vi "4Pi Objective Image Alignment.vi"(7 "Calling VI Ref":refnum<vi>) -> ()   [LabVIEW 2016]
uses:
  4Pi OIA - Controls/4Pi OIA - ROI Selection.ctl
  4Pi OIA - Controls/4Pi OIA - Method.ctl
  <vilib>/vision/Image Controls.llb/IMAQ Image.ctl
  4Pi OIA - Controls/4Pi OIA - Notifier Type.ctl
  4Pi OIA - Controls/4Pi OIA - Actions.ctl
  <vilib>/Utility/miscctls.llb/LVPointTypeDef.ctl
  Hardware Configuration/Hardware Configuration Controls/Device Function.ctl
  Hardware Configuration/Hardware Configuration Controls/Device Type.ctl
  Device Library/Cameras/Hamamatsu/Orca Flash/Orca Flash Controls/Orca Flash Actions.ctl
  Device Library/Shutters/Shutter Controls/Shutter Actions.ctl
  Device Library/Stages/Stages Controls/Stage Actions.ctl
  <resource>/objmgr/IMAQImage.rc
panel:
  in  "Alignment Cycles":u16=1 min=1 step=1
  in  "Get Shift":bool
  in  "Camera Px. Size (µm)":dbl=0.1 min=0.0 max=10.0
  in  "Frame Accums.":u16=1 min=1 step=1
  in  "Align":bool
  in  "Method":T1
  in  "Image Selection":i32(ring) items=["Quad 01", "Quad 02", "Quad 03", "Quad 04"]
  in  "ROI Selection":T2
  in  "Quit":bool
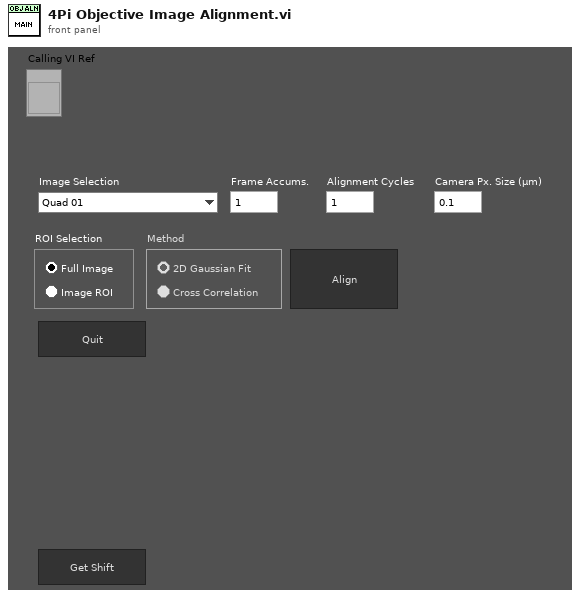
[diagram p1: front panel]
types:
  T1 = typedef "4Pi OIA - Method.ctl" = enum32{"2D Gaussian Fit", "Cross Correlation"}
  T2 = typedef "4Pi OIA - ROI Selection.ctl" = enum32{"Full Image", "ROI"}
  T3 = enum16{"Always On", "Always Off", "Off While Running"}
  T4 = typedef "LVPointTypeDef.ctl" = cluster{"Horizontal":i16, "Vertical":i16}
  T5 = typedef "4Pi OIA - Actions.ctl" = enum16{"Idle", "Start Alignment", "Get Upper Image", "Get Lower Image", "Get Shift", "Move OBJ", "Quit"}
  T6 = enum8{"Enabled", "Disabled", "Disabled and Grayed Out"}
  T7 = typedef "4Pi OIA - Notifier Type.ctl" = cluster{"Action":T5, "ROI Selection":T2, "Method":T1, "Frame Accums.":u16, "Camera Px. Size (µm)":dbl, "Image Ref":T8}
  T8 = typedef "IMAQ Image.ctl" = refnum<image>
  T9 = typedef "Device Function.ctl" = enum16{"Primary", "Secondary", "Overview", "Wide Field Drift Correction", "642 nm Excitation", "560 nm Excitation", "546 nm Excitation", "488 nm Excitation", "405 nm Excitation", "Objective Drift Correction", "Objective XY", "Objective Z", "Sample XY", "Sample Coarse Z", "Sample Z", "4Pi Lower", "4Pi Upper", "Adj Cavity"}
  T10 = typedef "Device Type.ctl" = enum16{"AOTF", "Camera", "Deformable Mirror", "Laser", "Shutter", "Stage"}
  T11 = typedef "Orca Flash Actions.ctl" = enum16{"IDLE", "PREVIEW", "RECORD", "Record Settings", "SETPARAM", "GETPARAM", "SETROI", "GETROI", "PROGRESSIVE MODE", "AREA MODE", "STATUS", "QUIT"}
  T12 = typedef "Shutter Actions.ctl" = enum16{"Open", "Close", "Toggle", "Status", "Quit"}
  T13 = typedef "Stage Actions.ctl" = enum16{"Get Position", "MVR", "MOVE", "HALT", "ONTARGET", "ERROR", "REFERENCE", "INIT", "VELOCITY", "STATUS", "EXIT", "HOME", "ZEROPOS", "NANOPOS", "ANALOG", "QUIT"}
  T14 = enum32{"Invalid", "Standard", "Closed", "Hidden", "Minimized", "Maximized"}
  T15 = typedef "2D Gaussian - Best Fit Parameters.ctl" = cluster{"Amplitude":dbl, "X Position":dbl, "Y Position":dbl, "X Width":dbl, "Y Width":dbl, "Offset":dbl}
  T16 = typedef "LVRectTypeDef.ctl" = cluster{"Left":i16, "Top":i16, "Right":i16, "Bottom":i16}
  T17 = typedef "LVBoundsTypeDef.ctl" = cluster{"Width":u32, "Height":u32}
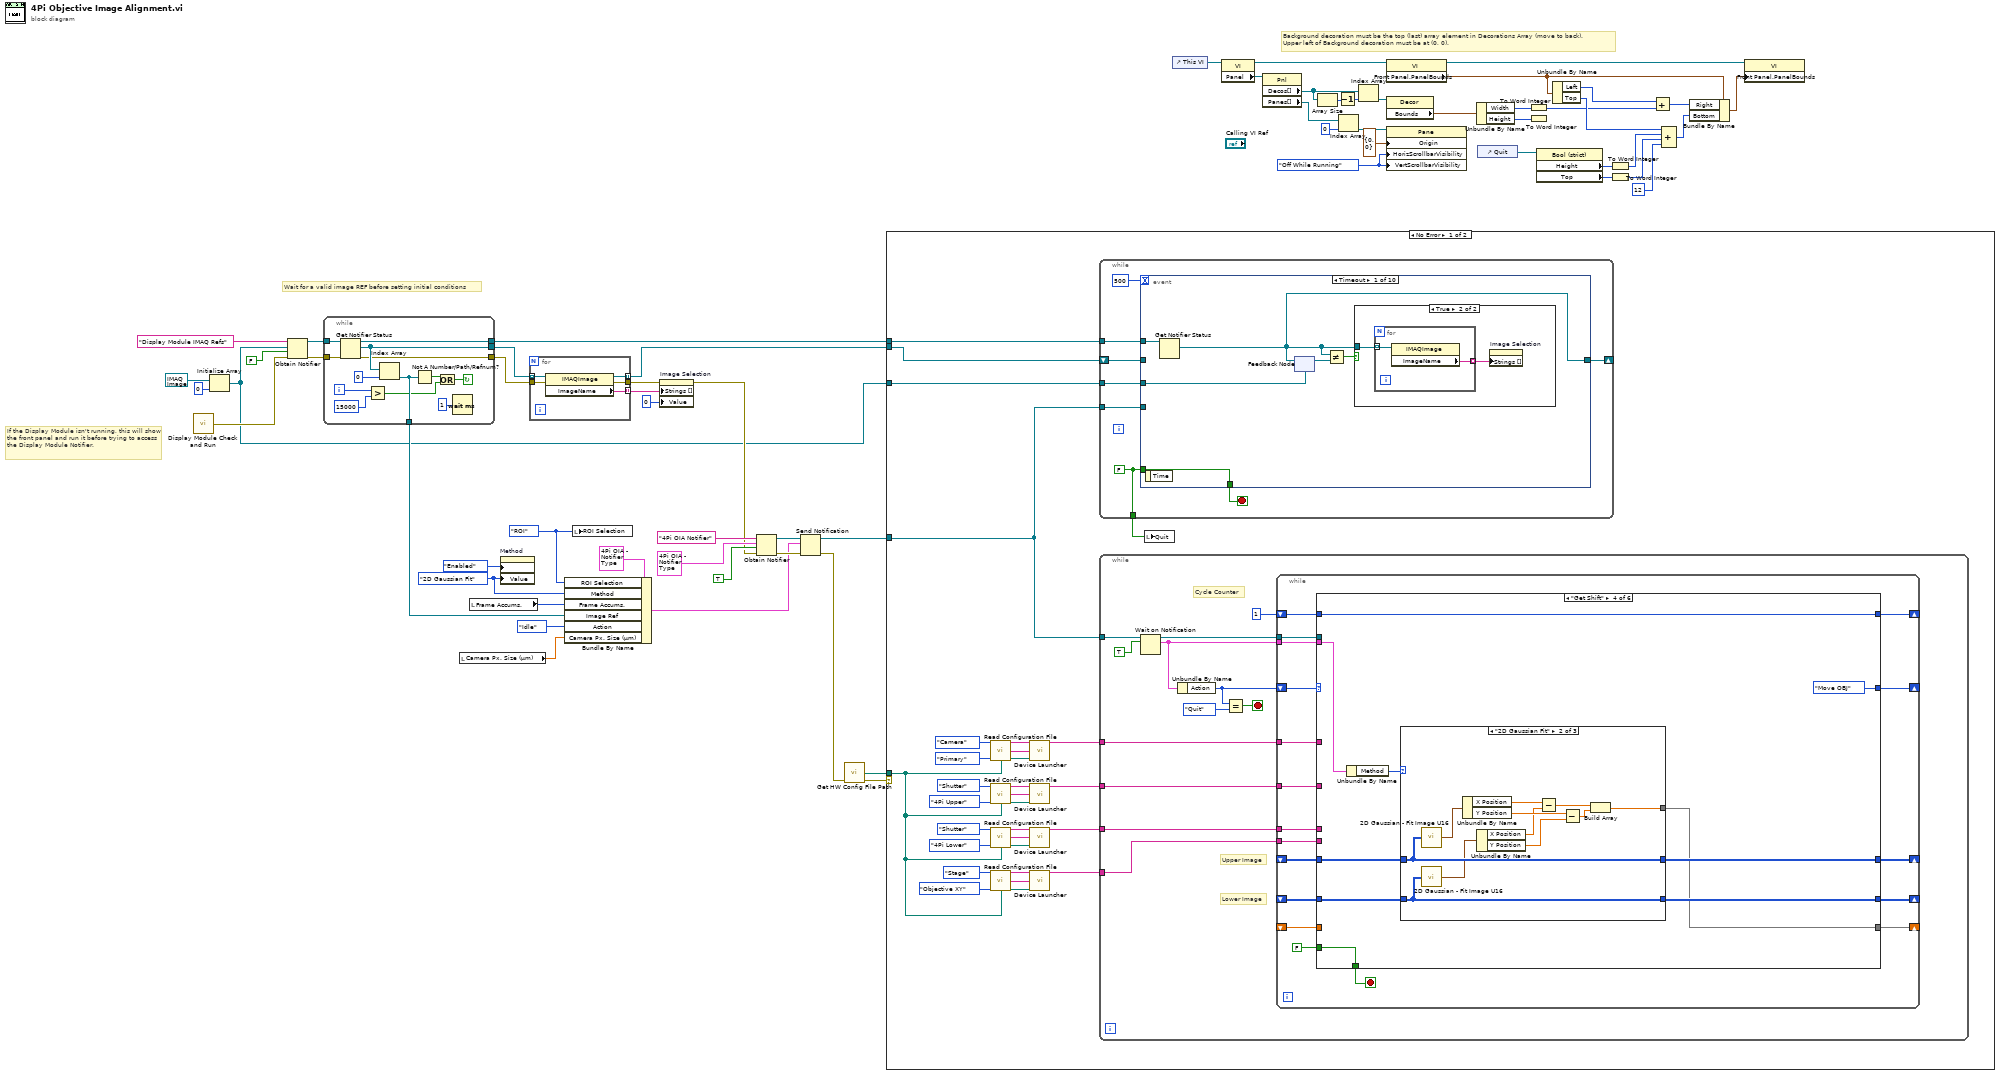
[diagram p0: block diagram]
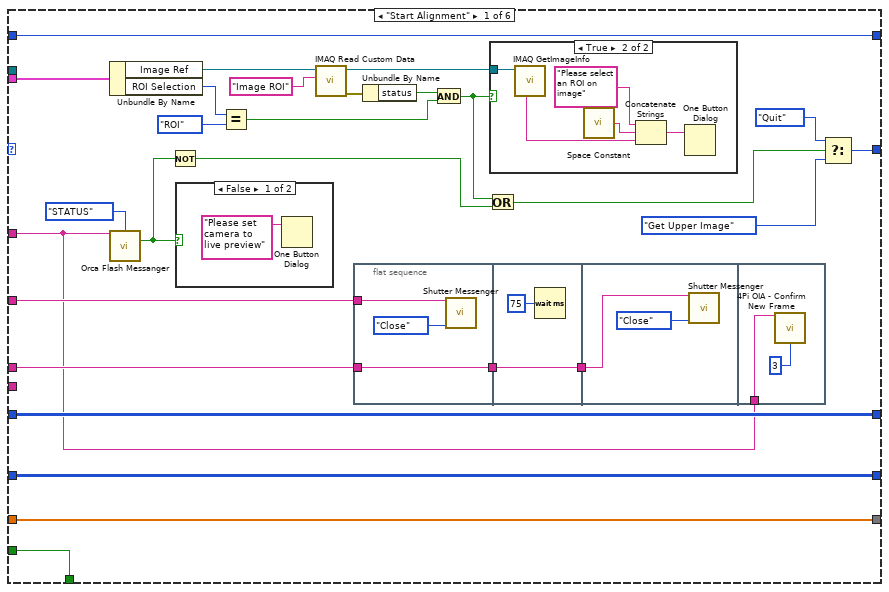
[diagram p2: hidden frame]
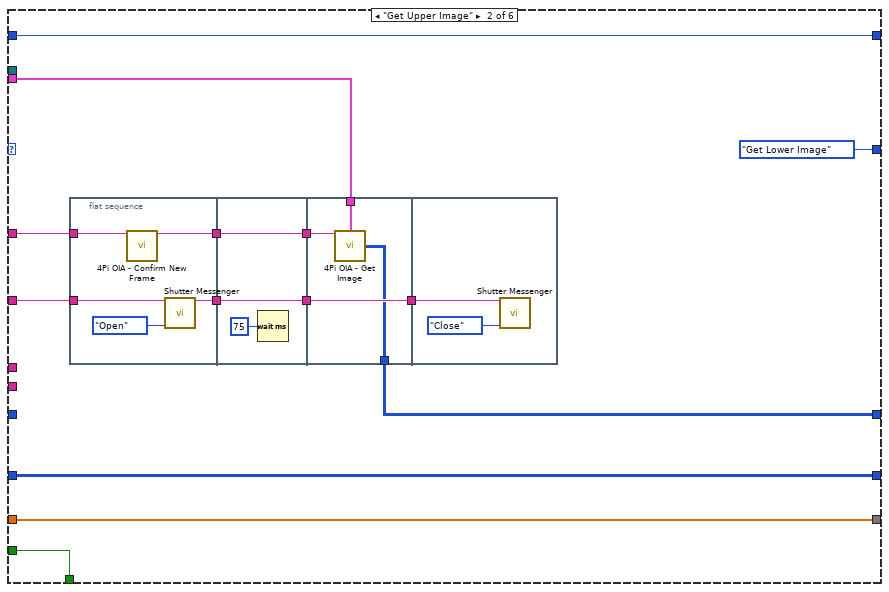
[diagram p5: hidden frame]
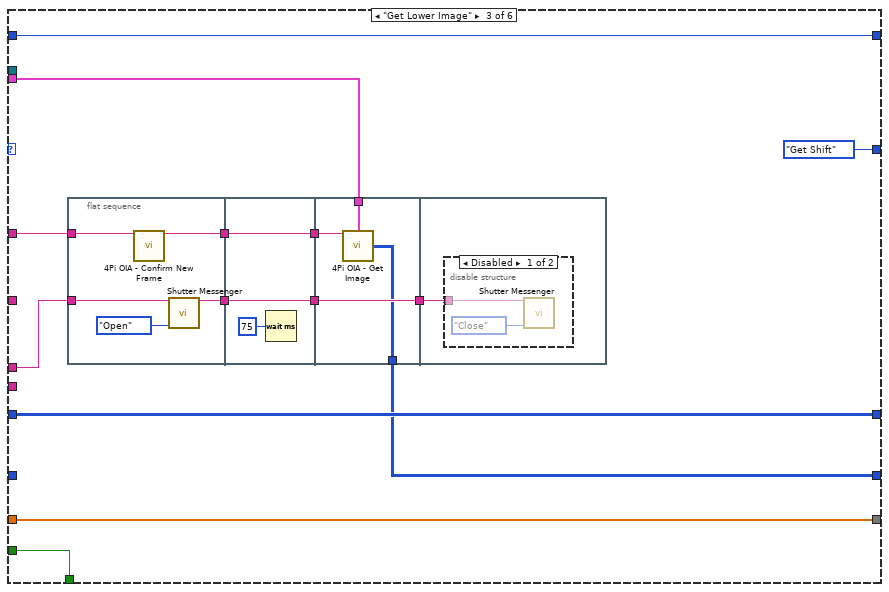
[diagram p6: hidden frame]
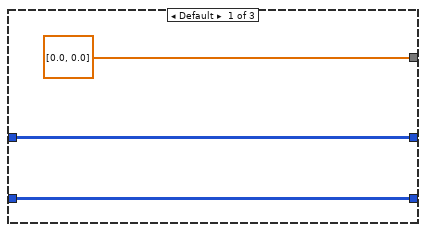
[diagram p8: hidden frame]
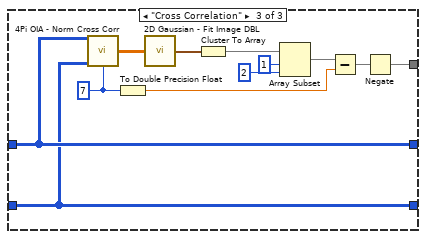
[diagram p9: hidden frame]
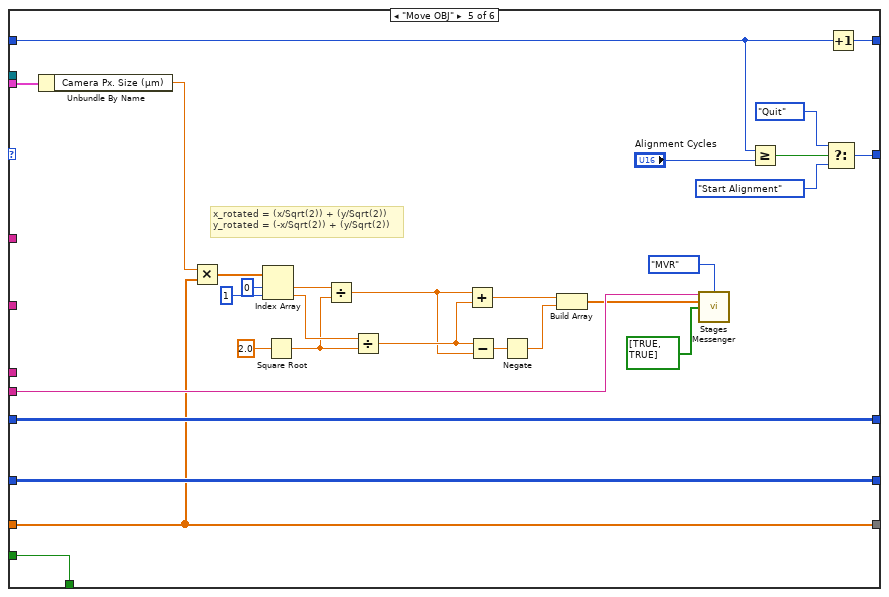
[diagram p10: hidden frame]
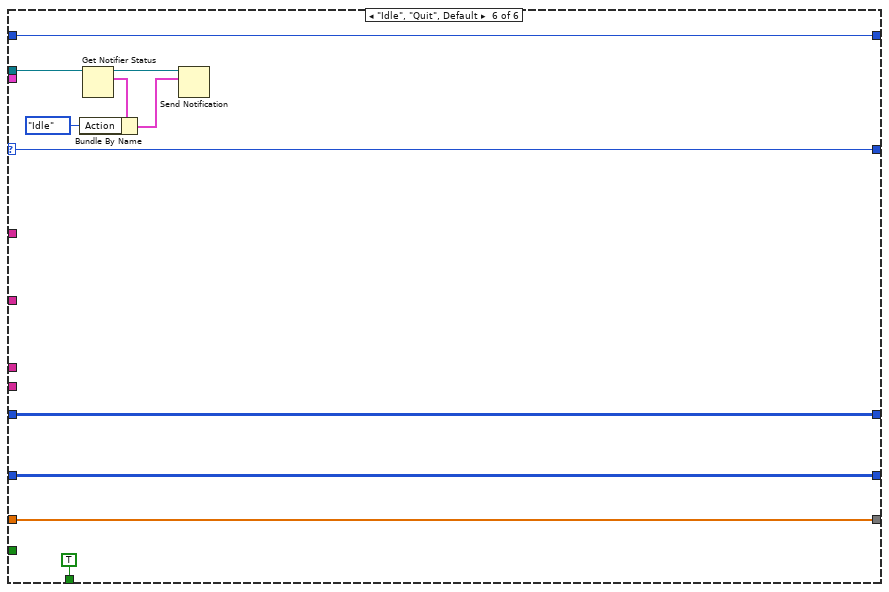
[diagram p11: hidden frame]
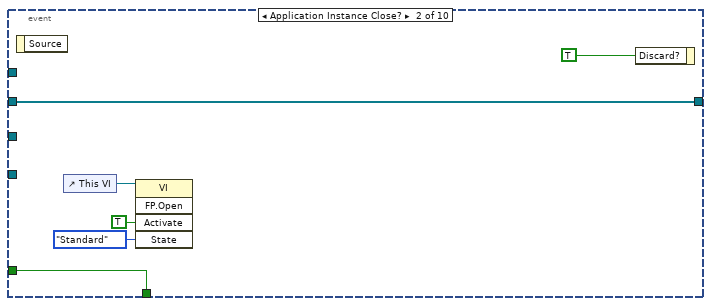
[diagram p13: hidden frame]
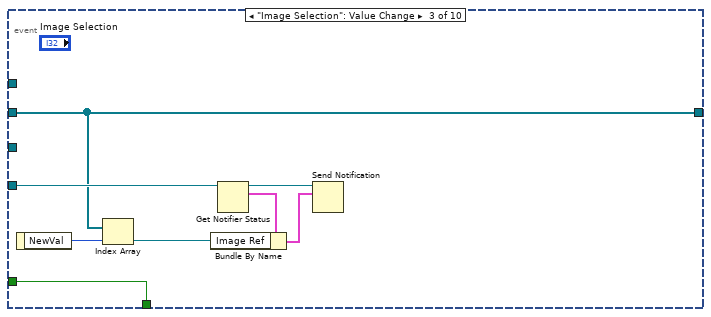
[diagram p14: hidden frame]
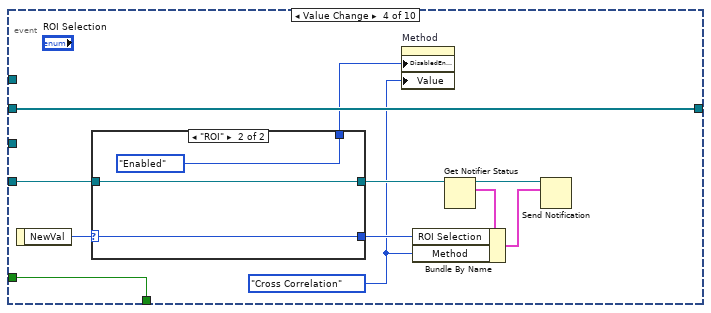
[diagram p15: hidden frame]
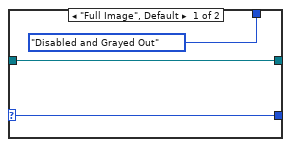
[diagram p16: hidden frame]
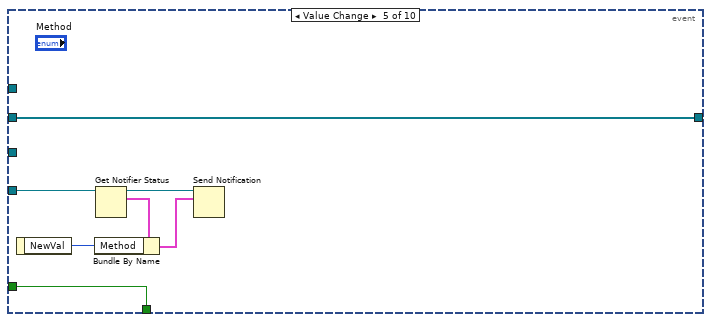
[diagram p17: hidden frame]
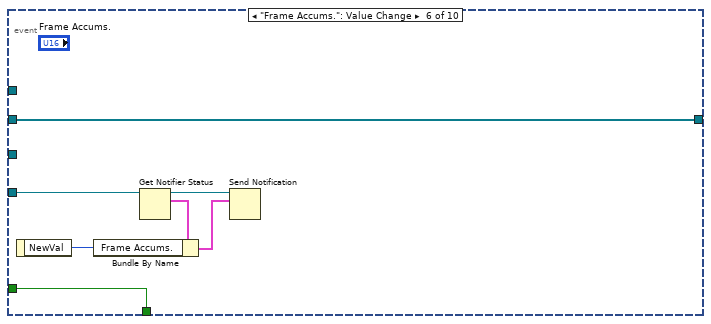
[diagram p18: hidden frame]
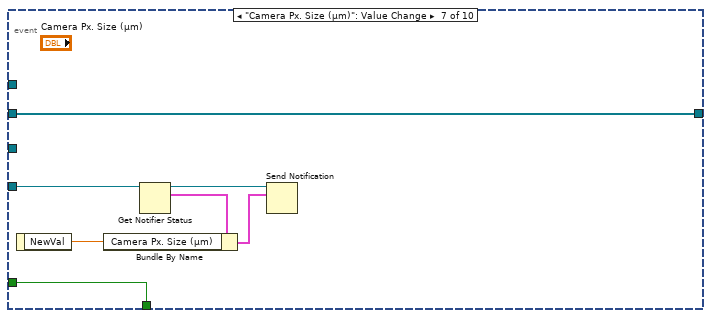
[diagram p19: hidden frame]
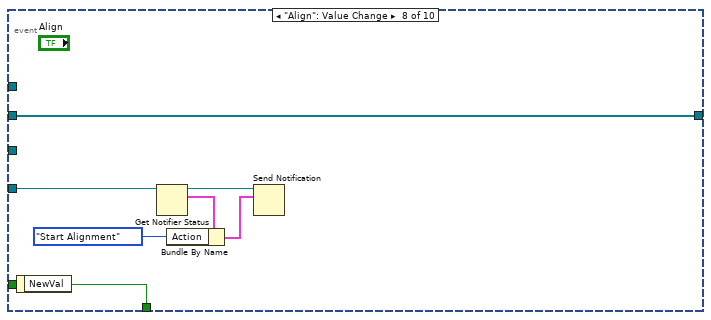
[diagram p20: hidden frame]
diagram:
  w25 = T3."Off While Running" ("Vertical Scrollbar Visibility")
  w51 = 4Pi_OIA_-_Method."2D Gaussian Fit" ("Method")
  w52 = 4Pi_OIA_-_ROI_Selection."ROI" ("ROI Selection")
  # "Wait for a valid image REF before setting initial conditions"
  # "If the Display Module isn't running, this will show the front panel and run it before trying to access the Display Module Notifier."
  # "Background decoration must be the top (last) array element in Decorations Array (move to back).\nUpper left of Background decoration must be at (0, 0)."
  n1 = call "Display Module Check and Run.vi"() -> ("Error"=w13:errorcluster)  [unwired: 15 in]
  n2 = Initialize Array(T8 refnum ("New Image"), 0 ("dimension size")) -> (w1:T8[])
  n3 = Obtain Notifier(name (unnamed)="Display Module IMAQ Refs", notification data type=w1, create if not found? (T)=FALSE, error in (no error)=w13) -> (notifier out=w12:refnum<notifier>, error out=w11:errorcluster)  [unwired: 1 out]
  n4 = while {
    tunnel: w12 -> [w76]
    tunnel: w11 -> [w75]
    tunnel: [w74] -> w10
    tunnel: [w73] -> w5
    tunnel: [w71] -> w9
    tunnel: [w69] -> w2
    i -> [w68]
    stop <- w65 continue-if-true
    n5 = Get Notifier Status(notifier=w76, error in (no error)=w75) -> (notifier out=w74:refnum<notifier>, current notification=w73:T8[], error out=w69:errorcluster)  [unwired: 2 out]
    n6 = Greater?(x=w68, y=15000) -> (0:w64:bool)
    n7 = Index Array(array=w73, index=0) -> (element=w71:T8)
    n8 = Not A Number/Path/Refnum?(number/path/refnum=w71) -> (NaN/Path/Refnum?=w66:bool)
    n9 = Or(x=w66, y=w64) -> (x .or. y?=w65:bool)
    n10 = Wait (ms)(milliseconds to wait=u32 1) -> ()  [unwired: 1 out]
  }
  n11 = local read "Camera Px. Size (µm)"() -> (w43:dbl)
  n12 = local read "Frame Accums."() -> (w45:u16)
  n13 = property on="Method" class="RadioBtnsControl (strict)"("DisabledEnum"=T6."Enabled" ("Disabled"), "Value"=w51) -> ()  [unwired: 2 in, 2 out]
  n14 = for {
    tunnel: w5 -> [w81] mode=indexing
    tunnel: [w80] -> w8 mode=indexing
    tunnel: [w79] -> w6
    tunnel: [w78] -> w4 mode=indexing
    tunnel: w2 -> [w77]
    n15 = property class="IMAQImage"(reference=w81, error in=w77) -> (reference out=w78:T8, error out=w79:errorcluster, "ImageName"=w80:string)
  }
  n16 = Bundle By Name(cluster=T7 {"Action"=enum."Start Alignment", "ROI Selection"=enum."Full Image", "Method"=enum."2D Gaussian Fit", "Frame Accums."=0, "Camera Px. Size (µm)"=0.0, "Image Ref"=refnum} ("4Pi OIA Notifier Type"), "ROI Selection"=w52, "Method"=w51, "Frame Accums."=w45, "Image Ref"=w9, "Action"=4Pi_OIA_-_Actions."Idle", "Camera Px. Size (µm)"=w43) -> (w47:T7)
  n17 = local write "ROI Selection"(w52) -> ()
  n18 = property on="Image Selection" class="Ring (strict)"(error in=w6, "Strings []"=w8, "Value"=0) -> (error out=w3:errorcluster)  [unwired: 1 in, 1 out]
  n19 = Obtain Notifier(name (unnamed)="4Pi OIA Notifier", notification data type=T7 {"Action"=enum."Start Alignment", "ROI Selection"=enum."Full Image", "Method"=enum."2D Gaussian Fit", "Frame Accums."=0, "Camera Px. Size (µm)"=0.0, "Image Ref"=refnum} ("4Pi OIA Notifier Type"), create if not found? (T)=TRUE, error in (no error)=w3) -> (notifier out=w50:refnum<notifier>, error out=w48:errorcluster)  [unwired: 1 out]
  n20 = Send Notification(notification=w47, notifier=w50, error in (no error)=w48) -> (notifier out=w49:refnum<notifier>, error out=w46:errorcluster)
  n21 = call "Get HW Config File Path.vi"("Error"=w46) -> ("File Path"=w62:path, "Error"=w63:errorcluster)  [unwired: 13 in]
  n22 = case shown="No Error" w63 {
    tunnel: w62 -> [w110 _]
    tunnel: w10 -> [w109 _]
    tunnel: w1 -> [w108 _]
    tunnel: w49 -> [w106 _]
    tunnel: w4 -> [w107 _]
    frame No Error {
      n23 = call "Read Configuration File.vi"("Device Type"=Device_Type."Camera", "Device Function"=Device_Function."Primary", "Config File Path"=w110) -> ("Unique Notifier Name"=w100:string, "Device Ports/IDs/Channels"=w102:string[], "Device Engine Path"=w101:path)  [unwired: 9 in, 1 out]
      n24 = call "Read Configuration File.vi"("Device Type"=Device_Type."Shutter", "Device Function"=Device_Function."4Pi Upper", "Config File Path"=w110) -> ("Unique Notifier Name"=w85:string, "Device Ports/IDs/Channels"=w87:string[], "Device Engine Path"=w86:path)  [unwired: 9 in, 1 out]
      n25 = call "Read Configuration File.vi"("Device Type"=Device_Type."Shutter", "Device Function"=Device_Function."4Pi Lower", "Config File Path"=w110) -> ("Unique Notifier Name"=w90:string, "Device Ports/IDs/Channels"=w88:string[], "Device Engine Path"=w89:path)  [unwired: 9 in, 1 out]
      n26 = call "Read Configuration File.vi"("Device Type"=Device_Type."Stage", "Device Function"=Device_Function."Objective XY", "Config File Path"=w110) -> ("Unique Notifier Name"=w95:string, "Device Ports/IDs/Channels"=w97:string[], "Device Engine Path"=w96:path)  [unwired: 9 in, 1 out]
      n27 = call "Device Launcher.vi"("Notifier Name"=w100, "Device Ports/IDs/Channels"=w102, "Device Engine Path"=w101) -> ("Notifier Name"=w105:string)  [unwired: 11 in, 1 out]
      n28 = call "Device Launcher.vi"("Notifier Name"=w85, "Device Ports/IDs/Channels"=w87, "Device Engine Path"=w86) -> ("Notifier Name"=w104:string)  [unwired: 11 in, 1 out]
      n29 = call "Device Launcher.vi"("Notifier Name"=w90, "Device Ports/IDs/Channels"=w88, "Device Engine Path"=w89) -> ("Notifier Name"=w103:string)  [unwired: 11 in, 1 out]
      n30 = call "Device Launcher.vi"("Notifier Name"=w95, "Device Ports/IDs/Channels"=w97, "Device Engine Path"=w96) -> ("Notifier Name"=w82:string)  [unwired: 11 in, 1 out]
      n31 = while {
        tunnel: [w322] -> w111
        tunnel: w109 -> [w321]
        tunnel: w108 -> [w320]
        tunnel: w106 -> [w319]
        shift-right: [w318] -> _
        shift-left: w107 -> [w317]
        stop <- w323 stop-if-true
        w322 = FALSE
        n32 = event shown="[0] Timeout" {
          selector: _ -> [_ _ _ _ _ _ _ _ _ _]
          dyn-events: _ -> [_ _ _ _ _ _ _ _ _ _]
          timeout: 500 -> [_ _ _ _ _ _ _ _ _ _]
          tunnel: w322 -> [w330 w339 w348 w358 w372 w379 w386 w393 w400 _]
          tunnel: [w330 w339 w348 w358 w372 w379 w386 w393 w400 w407] -> w323
          tunnel: w321 -> [w329 _ _ _ _ _ _ _ _ _]
          tunnel: w320 -> [w328 _ _ _ _ _ _ _ _ _]
          tunnel: w319 -> [_ _ w347 w353 w367 w374 w381 w392 w399 w401]
          tunnel: [w327 w335 w341 w359 w371 w378 w385 w387 w394 w406] -> w318
          tunnel: w317 -> [_ w335 w341 w359 w371 w378 w385 w387 w394 w406]
          event Timeout {
            n33 = event-data() -> ()  [unwired: 1 in, 1 out]
            n34 = Get Notifier Status(notifier=w329) -> (current notification=w327:T8[])  [unwired: 1 in, 4 out]
            n35 = feedback #1(w328) -> (w326:T8[])
            n36 = feedback-in #1(w327) -> ()
            n37 = Not Equal?(x=w327, y=w326) -> (x != y?=w325:bool)
            n38 = case shown="True" w325 {
              tunnel: w327 -> [_ w332]
              frame False {
              }
              frame True {
                n39 = for {
                  tunnel: w332 -> [w334] mode=indexing
                  tunnel: [w333] -> w331 mode=indexing
                  n40 = property class="IMAQImage"(reference=w334) -> ("ImageName"=w333:string)  [unwired: 1 in, 2 out]
                }
                n41 = property on="Image Selection" class="Ring (strict)"("Strings []"=w331) -> ()  [unwired: 2 in, 2 out]
              }
            }
          }
          event Application Instance Close? {
            n42 = event-data() -> ()  [unwired: 1 in, 1 out]
            n43 = control-ref of="This VI"() -> (w336:refnum<vi>)
            n44 = invoke class="VI" method="FP.Open"(reference=w336, "Activate"=TRUE ("Activate?"), "State"=T14."Standard") -> ()  [unwired: 2 in, 5 out]
            n45 = event-data("Discard?"=TRUE) -> ()  [unwired: 1 in, 1 out]
          }
          event "Image Selection": Value Change {
            n46 = event-data() -> ("NewVal"=w343:i32)  [unwired: 1 in]
            n47 = Index Array(array=w341, index=w343) -> (element=w342:T8)
            n48 = Get Notifier Status(notifier=w347) -> (notifier out=w346:refnum<notifier>, current notification=w345:T7)  [unwired: 1 in, 3 out]
            n49 = Bundle By Name(cluster=w345, "Image Ref"=w342) -> (w344:T7)
            n50 = Send Notification(notification=w344, notifier=w346) -> ()  [unwired: 1 in, 2 out]
          }
          event Value Change {
            w349 = 4Pi_OIA_-_Method."Cross Correlation" ("Method")
            n51 = event-data() -> ("NewVal"=w354:T2)  [unwired: 1 in]
            n52 = case shown="\"ROI\"" w354 {
              selector: w354 -> [w362 w364]
              tunnel: w353 -> [w361 w365]
              tunnel: [w362 w364] -> w351
              tunnel: [w361 w365] -> w352
              tunnel: [T6."Disabled and Grayed Out" ("Disabled") T6."Enabled" ("Disabled")] -> w350
              frame "Full Image", Default {
              }
              frame "ROI" {
              }
            }
            n53 = property on="Method" class="RadioBtnsControl (strict)"("DisabledEnum"=w350, "Value"=w349) -> ()  [unwired: 2 in, 2 out]
            n54 = Get Notifier Status(notifier=w352) -> (notifier out=w357:refnum<notifier>, current notification=w356:T7)  [unwired: 1 in, 3 out]
            n55 = Bundle By Name(cluster=w356, "ROI Selection"=w351, "Method"=w349) -> (w355:T7)
            n56 = Send Notification(notification=w355, notifier=w357) -> ()  [unwired: 1 in, 2 out]
          }
          event Value Change {
            n57 = event-data() -> ("NewVal"=w366:T1)  [unwired: 1 in]
            n58 = Get Notifier Status(notifier=w367) -> (notifier out=w370:refnum<notifier>, current notification=w369:T7)  [unwired: 1 in, 3 out]
            n59 = Bundle By Name(cluster=w369, "Method"=w366) -> (w368:T7)
            n60 = Send Notification(notification=w368, notifier=w370) -> ()  [unwired: 1 in, 2 out]
          }
          event "Frame Accums.": Value Change {
            n61 = event-data() -> ("NewVal"=w373:u16)  [unwired: 1 in]
            n62 = Get Notifier Status(notifier=w374) -> (notifier out=w377:refnum<notifier>, current notification=w376:T7)  [unwired: 1 in, 3 out]
            n63 = Bundle By Name(cluster=w376, "Frame Accums."=w373) -> (w375:T7)
            n64 = Send Notification(notification=w375, notifier=w377) -> ()  [unwired: 1 in, 2 out]
          }
          event "Camera Px. Size (µm)": Value Change {
            n65 = event-data() -> ("NewVal"=w380:dbl)  [unwired: 1 in]
            n66 = Get Notifier Status(notifier=w381) -> (notifier out=w384:refnum<notifier>, current notification=w383:T7)  [unwired: 1 in, 3 out]
            n67 = Bundle By Name(cluster=w383, "Camera Px. Size (µm)"=w380) -> (w382:T7)
            n68 = Send Notification(notification=w382, notifier=w384) -> ()  [unwired: 1 in, 2 out]
          }
          event "Align": Value Change {
            n69 = event-data() -> ()  [unwired: 1 in, 1 out]
            n70 = Get Notifier Status(notifier=w392) -> (notifier out=w391:refnum<notifier>, current notification=w390:T7)  [unwired: 1 in, 3 out]
            n71 = Bundle By Name(cluster=w390, "Action"=4Pi_OIA_-_Actions."Start Alignment") -> (w389:T7)
            n72 = Send Notification(notification=w389, notifier=w391) -> ()  [unwired: 1 in, 2 out]
          }
          event "Get Shift": Value Change {
            # "For debugging only"
            n73 = event-data() -> ()  [unwired: 1 in, 1 out]
            n74 = Get Notifier Status(notifier=w399) -> (notifier out=w398:refnum<notifier>, current notification=w397:T7)  [unwired: 1 in, 3 out]
            n75 = Bundle By Name(cluster=w397, "Action"=4Pi_OIA_-_Actions."Get Shift") -> (w396:T7)
            n76 = Send Notification(notification=w396, notifier=w398) -> ()  [unwired: 1 in, 2 out]
          }
          event "Quit": Value Change {
            n77 = event-data() -> ("NewVal"=w407:bool)  [unwired: 1 in]
            n78 = Get Notifier Status(notifier=w401) -> (notifier out=w402:refnum<notifier>, current notification=w403:T7)  [unwired: 1 in, 3 out]
            n79 = Bundle By Name(cluster=w403, "Action"=4Pi_OIA_-_Actions."Quit") -> (w404:T7)
            n80 = Send Notification(notification=w404, notifier=w402) -> ()  [unwired: 1 in, 2 out]
          }
        }
      }
      n81 = while {
        tunnel: w106 -> [w123]
        tunnel: w105 -> [w118]
        tunnel: w104 -> [w117]
        tunnel: w103 -> [w116]
        tunnel: w82 -> [w113]
        stop <- w120 stop-if-true
        # "Cycle Counter"
        # "Lower Image"
        # "Upper Image"
        n82 = Wait on Notification(notifier=w123, ignore previous (F)=TRUE) -> (notifier out=w114:refnum<notifier>, notification=w115:T7)  [unwired: 2 in, 2 out]
        n83 = Unbundle By Name(w115) -> ("Action"=w119:T5)
        n84 = Equal?(x=w119, y=4Pi_OIA_-_Actions."Quit") -> (x = y?=w120:bool)
        n85 = while {
          shift-right: [w138] -> _
          shift-left: w119 -> [w141]
          tunnel: w118 -> [w137]
          tunnel: w117 -> [w136]
          tunnel: w116 -> [w135]
          shift-right: [w132] -> _
          shift-left: _ -> [w131]
          shift-right: [w134] -> _
          shift-left: _ -> [w133]
          tunnel: w115 -> [w130]
          tunnel: w114 -> [w129]
          tunnel: w113 -> [w128]
          shift-right: [w127] -> _
          shift-left: _ -> [w126]
          shift-right: [w124] -> _
          shift-left: u16 1 -> [w125]
          stop <- w139 stop-if-true
          n86 = case shown="\"Get Shift\"" w141 {
            selector: w141 -> [_ _ _ _ _ w315]
            tunnel: FALSE -> [w168 w196 w224 w249 w305 _]
            tunnel: [w168 w196 w224 w249 w305 TRUE] -> w139
            tunnel: [w153 4Pi_OIA_-_Actions."Get Lower Image" ("Action") 4Pi_OIA_-_Actions."Get Shift" ("Action") 4Pi_OIA_-_Actions."Move OBJ" ("Action") w279 w315] -> w138
            tunnel: w137 -> [w145 w187 w218 _ _ _]
            tunnel: w136 -> [w151 w195 _ _ _ _]
            tunnel: w135 -> [w150 _ w215 _ _ _]
            tunnel: [w147 w189 w216 w243 w303 w313] -> w134
            tunnel: w133 -> [w147 w189 _ w245 w303 w313]
            tunnel: [w146 w188 w217 w244 w304 w314] -> w132
            tunnel: w131 -> [w146 _ w217 w246 w304 w314]
            tunnel: w130 -> [w144 w186 w214 w247 w299 _]
            tunnel: w129 -> [_ _ _ _ _ w308]
            tunnel: w128 -> [_ _ _ _ w302 _]
            tunnel: [w143 w185 w213 w242 w287 w307] -> w127
            tunnel: w126 -> [w143 w185 w213 _ w287 w307]
            tunnel: w125 -> [w142 w184 w212 w241 w278 w306]
            tunnel: [w142 w184 w212 w241 w277 w306] -> w124
            frame "Start Alignment" {
              n87 = Unbundle By Name(w144) -> ("Image Ref"=w165:T8, "ROI Selection"=w167:T2)
              n88 = call "Orca Flash Messanger.vi"("Notifier Name"=w145, "Camera Actions"=Orca_Flash_Actions."STATUS") -> ("Running?"=w157:bool)  [unwired: 9 in, 4 out]
              n89 = Not(x=w157) -> (.not. x?=w156:bool)
              n90 = case shown="False" w157 {
                frame False {
                  n91 = One Button Dialog(message="Please set camera to live preview") -> ()  [unwired: 1 in, 1 out]
                }
                frame True {
                }
              }
              n92 = Equal?(x=w167, y=4Pi_OIA_-_ROI_Selection."ROI") -> (x = y?=w161:bool)
              n93 = call "IMAQ Read Custom Data"("Key"="Image ROI", "Image"=w165) -> ("error out"=w163:errorcluster, "Image (duplicate)"=w160:T8)  [unwired: 7 in, 1 out]
              n94 = flat-sequence {
                tunnel: w151 -> [w170]
                tunnel: w150 -> [w169]
                tunnel: [w169] -> w149
                tunnel: w149 -> [w173]
                tunnel: [w173] -> w148
                tunnel: w148 -> [w174]
                tunnel: w145 -> [w177]
                frame #0 {
                  n95 = call "Shutter Messenger.vi"("Notifier Name"=w170, "Action"=Shutter_Actions."Close") -> ()  [unwired: 12 in, 2 out]
                }
                frame #1 {
                  n96 = Wait (ms)(milliseconds to wait=u32 75) -> ()  [unwired: 1 out]
                }
                frame #2 {
                  n97 = call "Shutter Messenger.vi"("Notifier Name"=w174, "Action"=Shutter_Actions."Close") -> ()  [unwired: 12 in, 2 out]
                }
                frame #3 {
                  n98 = call "4Pi OIA - Confirm New Frame.vi"("Camera Notifier Name"=w177, "Wait No. (1)"=u32 3 ("Wait No.")) -> ()  [unwired: 13 in, 1 out]
                }
              }
              n99 = Unbundle By Name(w163) -> ("status"=w162:bool)
              n100 = And(x=w162, y=w161) -> (x .and. y?=w158:bool)
              n101 = Or(x=w158, y=w156) -> (x .or. y?=w155:bool)
              n102 = case shown="True" w158 {
                tunnel: w160 -> [_ w183]
                frame False {
                }
                frame True {
                  n103 = call "IMAQ GetImageInfo"("Image"=w183) -> ("Image Name"=w182:string)  [unwired: 3 in, 7 out]
                  n104 = call <vilib>:"Space Constant.vi"() -> ("String"=w181:string)
                  n105 = Concatenate Strings("Please select an ROI on image", w181, w182) -> (w179:string)
                  n106 = One Button Dialog(message=w179) -> ()  [unwired: 1 in, 1 out]
                }
              }
              n107 = Select(t=4Pi_OIA_-_Actions."Quit" ("Action"), s=w155, f=4Pi_OIA_-_Actions."Get Upper Image") -> (s? t:f=w153:T5)
            }
            frame "Get Upper Image" {
              n108 = flat-sequence {
                tunnel: [w200] -> w192
                tunnel: [w198] -> w190
                tunnel: w195 -> [w201]
                tunnel: w187 -> [w199]
                tunnel: [w205] -> w193
                tunnel: w192 -> [w205]
                tunnel: [w203] -> w191
                tunnel: w190 -> [w203]
                tunnel: [w209] -> w194
                tunnel: w193 -> [w209]
                tunnel: w191 -> [w208]
                tunnel: w186 -> [w207]
                tunnel: [w206] -> w188
                tunnel: w194 -> [w210]
                frame #0 {
                  n109 = call "4Pi OIA - Confirm New Frame.vi"("Camera Notifier Name"=w199) -> ("Camera Notifier Name (Dup)"=w198:string)  [unwired: 14 in]
                  n110 = call "Shutter Messenger.vi"("Notifier Name"=w201, "Action"=Shutter_Actions."Open") -> ("Notifier Name Dup"=w200:string)  [unwired: 12 in, 1 out]
                }
                frame #1 {
                  n111 = Wait (ms)(milliseconds to wait=u32 75) -> ()  [unwired: 1 out]
                }
                frame #2 {
                  n112 = call "4Pi OIA - Get Image.vi"("Camera Notifier Name"=w208, "Alignment Data"=w207) -> ("Image Out"=w206:u16[][])  [unwired: 13 in]
                }
                frame #3 {
                  n113 = call "Shutter Messenger.vi"("Notifier Name"=w210, "Action"=Shutter_Actions."Close") -> ()  [unwired: 12 in, 2 out]
                }
              }
            }
            frame "Get Lower Image" {
              n114 = flat-sequence {
                tunnel: [w229] -> w221
                tunnel: [w226] -> w219
                tunnel: w218 -> [w227]
                tunnel: w215 -> [w228]
                tunnel: [w233] -> w222
                tunnel: w221 -> [w233]
                tunnel: [w231] -> w220
                tunnel: w219 -> [w231]
                tunnel: [w237] -> w223
                tunnel: w222 -> [w237]
                tunnel: w220 -> [w236]
                tunnel: w214 -> [w235]
                tunnel: [w234] -> w216
                tunnel: w223 -> [w238]
                frame #0 {
                  n115 = call "4Pi OIA - Confirm New Frame.vi"("Camera Notifier Name"=w227) -> ("Camera Notifier Name (Dup)"=w226:string)  [unwired: 14 in]
                  n116 = call "Shutter Messenger.vi"("Notifier Name"=w228, "Action"=Shutter_Actions."Open") -> ("Notifier Name Dup"=w229:string)  [unwired: 12 in, 1 out]
                }
                frame #1 {
                  n117 = Wait (ms)(milliseconds to wait=u32 75) -> ()  [unwired: 1 out]
                }
                frame #2 {
                  n118 = call "4Pi OIA - Get Image.vi"("Camera Notifier Name"=w236, "Alignment Data"=w235) -> ("Image Out"=w234:u16[][])  [unwired: 13 in]
                }
                frame #3 {
                  n119 = disable-structure shown="Disabled" {
                    disable-tunnel: w238 -> [w239 _]
                    frame Disabled {
                      n120 = call "Shutter Messenger.vi"("Notifier Name"=w239, "Action"=Shutter_Actions."Close") -> ()  [unwired: 12 in, 2 out]
                    }
                    frame Enabled {
                    }
                  }
                }
              }
            }
            frame "Get Shift" {
              n121 = Unbundle By Name(w247) -> ("Method"=w248:T1)
              n122 = case shown="\"2D Gaussian Fit\"" w248 {
                tunnel: w246 -> [w253 w264 w276]
                tunnel: w245 -> [w252 w263 w275]
                tunnel: [w253 w264 w276] -> w244
                tunnel: [w252 w263 w275] -> w243
                tunnel: [dbl[] [0.0, 0.0] w255 w265] -> w242
                frame Default {
                }
                frame "2D Gaussian Fit" {
                  n123 = call "2D Gaussian - Fit Image U16.vi"("Image In (U16)"=w264) -> ("Best Fit Params"=w254:T15)  [unwired: 14 in]
                  n124 = call "2D Gaussian - Fit Image U16.vi"("Image In (U16)"=w263) -> ("Best Fit Params"=w262:T15)  [unwired: 14 in]
                  n125 = Unbundle By Name(w254) -> ("X Position"=w261:dbl, "Y Position"=w260:dbl)
                  n126 = Unbundle By Name(w262) -> ("X Position"=w259:dbl, "Y Position"=w258:dbl)
                  n127 = Subtract(x=w261, y=w259) -> (x-y=w257:dbl)
                  n128 = Subtract(x=w260, y=w258) -> (x-y=w256:dbl)
                  n129 = Build Array(w257, w256) -> (w255:dbl[])
                }
                frame "Cross Correlation" {
                  w269 = 7 ("Half Shift")
                  n130 = call "4Pi OIA - Norm Cross Corr.vi"("Image 01"=w276, "Image 02"=w275, "Half Shift"=w269) -> ("Norm Cross Corr Result"=w274:dbl[][])  [unwired: 12 in]
                  n131 = To Double Precision Float(number=w269) -> (double precision float=w267:dbl)
                  n132 = call "2D Gaussian - Fit Image DBL.vi"("Image In (DBL)"=w274) -> ("Best Fit Params"=w273:T15)  [unwired: 14 in]
                  n133 = Cluster To Array(cluster=w273) -> (array=w272:dbl[])
                  n134 = Array Subset(array=w272, index=1, length=2) -> (w268:dbl[])
                  n135 = Subtract(x=w268, y=w267) -> (x-y=w266:dbl[])
                  n136 = Negate(x=w266) -> (-x=w265:dbl[])
                }
              }
            }
            frame "Move OBJ" {
              # "x_rotated = (x/Sqrt(2)) + (y/Sqrt(2))\ny_rotated = (-x/Sqrt(2)) + (y/Sqrt(2))"
              n137 = Unbundle By Name(w299) -> ("Camera Px. Size (µm)"=w285:dbl)
              n138 = Multiply(x=w285, y=w287) -> (x*y=w286:dbl[])
              n139 = Index Array(array=w286, index #1=0 ("index"), index #2=1 ("index")) -> (element #1=w296:dbl, element #2=w294:dbl)
              n140 = Square Root(x=2.0) -> (sqrt(x)=w293:dbl)
              n141 = Divide(x=w296, y=w293) -> (x/y=w291:dbl)
              n142 = Divide(x=w294, y=w293) -> (x/y=w292:dbl)
              n143 = Add(x=w291, y=w292) -> (x+y=w284:dbl)
              n144 = Subtract(x=w292, y=w291) -> (x-y=w289:dbl)
              n145 = Negate(x=w289) -> (-x=w288:dbl)
              n146 = Build Array(w284, w288) -> (w290:dbl[])
              n147 = call "Stages Messenger.vi"("Stage Notifier Name"=w302, "Actions"=Stage_Actions."MVR", "Setpoint"=w290, "Axis"=bool[] [TRUE, TRUE]) -> ()  [unwired: 8 in, 4 out]
              n148 = Greater Or Equal?(x=w278, y="Alignment Cycles") -> (x >= y?=w280:bool)
              n149 = Select(t=4Pi_OIA_-_Actions."Quit" ("Action"), s=w280, f=4Pi_OIA_-_Actions."Start Alignment" ("Action")) -> (s? t:f=w279:T5)
              n150 = Increment(x=w278) -> (x+1=w277:u16)
            }
            frame "Idle", "Quit", Default {
              n151 = Get Notifier Status(notifier=w308) -> (notifier out=w312:refnum<notifier>, current notification=w311:T7)  [unwired: 1 in, 3 out]
              n152 = Bundle By Name(cluster=w311, "Action"=4Pi_OIA_-_Actions."Idle") -> (w310:T7)
              n153 = Send Notification(notification=w310, notifier=w312) -> ()  [unwired: 1 in, 2 out]
            }
          }
        }
      }
      n154 = local write "Quit"(w111) -> ()
    }
    frame Error {
      n155 = One Button Dialog(message="Objective image alignment tool failed to start.") -> ()  [unwired: 1 in, 1 out]
    }
  }
  n156 = control-ref of="This VI"() -> (w17:refnum<vi>)
  n157 = property class="VI"(reference=w17) -> (reference out=w26:refnum<vi>, "Panel"=w18:refnum<vi>)  [unwired: 1 in, 1 out]
  n158 = property class="Pnl"(reference=w18) -> ("Decos[]"=w16:refnum<vi>[], "Panes[]"=w22:refnum<vi>[])  [unwired: 1 in, 2 out]
  n159 = Array Size(array=w16) -> (size(s)=w14:i32)
  n160 = Decrement(x=w14) -> (x-1=w15:i32)
  n161 = Index Array(array=w22, index=0) -> (element=w21:refnum<vi>)
  n162 = Index Array(array=w16, index=w15) -> (element=w24:refnum<vi>)
  n163 = property class="VI"(reference=w26) -> (reference out=w28:refnum<vi>, "Front Panel.PanelBounds"=w29:T16)  [unwired: 1 in, 1 out]
  n164 = property class="Decor"(reference=w24) -> ("Bounds"=w27:T17)  [unwired: 1 in, 2 out]
  n165 = property class="Pane"(reference=w21, "Origin"=T4 {"Horizontal"=0, "Vertical"=0}, "HorizScrollbarVisibility"=w25, "VertScrollbarVisibility"=w25) -> ()  [unwired: 1 in, 2 out]
  n166 = Unbundle By Name(w27) -> ("Width"=w32:u32, "Height"=w35:u32)
  n167 = control-ref of="Quit"() -> (w19:refnum<vi>)
  n168 = To Word Integer(number=w32) -> (16bit integer=w34:i16)
  n169 = To Word Integer(number=w35) -> ()  [unwired: 1 out]
  n170 = property class="Bool (strict)"(reference=w19) -> ("Height"=w37:u32, "Top"=w38:i32)  [unwired: 1 in, 2 out]
  n171 = Unbundle By Name(w29) -> ("Left"=w31:i16, "Top"=w42:i16)
  n172 = To Word Integer(number=w37) -> (16bit integer=w40:i16)
  n173 = To Word Integer(number=w38) -> (16bit integer=w41:i16)
  n174 = Add(x=w31, y=w34) -> (x+y=w33:i16)
  n175 = Compound Arithmetic op=ADD(w42, w40, w41, i16 12 ("y")) -> (w36:i16)
  n176 = Bundle By Name(cluster=w29, "Right"=w33, "Bottom"=w36) -> (w30:T16)
  n177 = property class="VI"(reference=w28, "Front Panel.PanelBounds"=w30) -> ()  [unwired: 1 in, 2 out]
